vi "allSettings.vi"() -> ()   [LabVIEW 2018]
panel:
  in  "Additional Commands":T1={"Read/Write RAM"={"Dictionary Name"="Enable/Disable Channel", "Dictionary ID"="41", "Update"=FALSE, "Current Data"=""}, "Set/Read Address Pointer"={"Dictionary Name"="Set/Read address pointer", "Dictionary ID"="40", "Update"=FALSE, "Current Data"=""}, "Read EE chksm"={"Dictionary Name"="Read EEPROM Checksum", "Dictionary ID"="42", "Update"=FALSE, "Current Data"=""}, "Hold On/Off"={"Dictionary Name"="Hold On/Off", "Dictionary ID"="43", "Update"=FALSE, "Current Data"=""}, "Emulator Mode"={"Dictionary Name"="Set/Reset Emulator Mode", "Dictionary ID"="44", "Update"=FALSE, "Current Data"=""}, "Write Protect Signal"={"Dictionary Name"="Write Protect Signal On/Off", "Dictionary ID"="45", "Update"=FALSE, "Current Data"=""}}
  in  "Channel Commands":T2={"Chan number"={"Dictionary Name"="Set/Read Channel Number", "Dictionary ID"="30", "Update"=FALSE, "Current Data"=""}, "En/Dis Channel"={"Dictionary Name"="Enable/Disable Channel", "Dictionary ID"="31", "Update"=FALSE, "Current Data"=""}}
  in  "Info Commands":T3={"Part Num"={"Dictionary Name"="Read Part Number", "Dictionary ID"="10", "Update"=FALSE, "Current Data"=""}, "Serial Num"={"Dictionary Name"="Read Part Number", "Dictionary ID"="11", "Update"=FALSE, "Current Data"=""}, "F/W Ver"={"Dictionary Name"="Read F/W & Module Version", "Dictionary ID"="12", "Update"=FALSE, "Current Data"=""}, "Status Byte"={"Dictionary Name"="Read Status Byte", "Dictionary ID"="13", "Update"=FALSE, "Ready/Busy"=FALSE, "Data in FIFO?"=FALSE, "FIFO Full?"=FALSE, "Event Mode On?"=FALSE, "GPIO I/P State"=FALSE, "Parity Error"=FALSE}, "Temp"={"Dictionary Name"="Read Temperature", "Dictionary ID"="14", "Update"=FALSE, "Current Data"=""}}
  in  "C&C Commands":T4={"Send Break"={"Dictionary Name"="Send Break Command", "Dictionary ID"="20", "Update"=FALSE, "Current Data"=""}, "Clear FIFO"={"Dictionary Name"="Clear Event FIFO", "Dictionary ID"="21", "Update"=FALSE, "Current Data"=""}, "Event Mode ON/OFF"={"Dictionary Name"="Event Mode On/Off", "Dictionary ID"="22", "Update"=FALSE, "Current Data"=""}, "Set Energy Threshold"={"Dictionary Name"="Set/Read Energy Threshold", "Dictionary ID"="23", "Update"=FALSE, "Current Data"=""}, "Set GPIO Mode"={"Dictionary Name"="Set/Read GPIO Signal Mode", "Dictionary ID"="24", "Update"=FALSE, "Current Data"=""}, "R/W Clock Freq"={"Dictionary Name"="Read/Write Clock Frequency", "Dictionary ID"="25", "Update"=FALSE, "Current Data"=""}, "Update/Restore Setup"={"Dictionary Name"="Update/Restore Setup", "Dictionary ID"="26", "Update"=FALSE, "Current Data"=""}, "Update/Read Peaking Time"={"Dictionary Name"="Update/Read Peaking Time", "Dictionary ID"="27", "Update"=FALSE, "Current Data"=""}, "Run/Read Self Test"={"Dictionary Name"="Run Self test/ Read Results", "Dictionary ID"="28", "Update"=FALSE, "Current Data"=""}}
  # "Additional Commands"
  # "Channel Commands"
  # "Information Commands"
  # "Configuration & Control Commands"
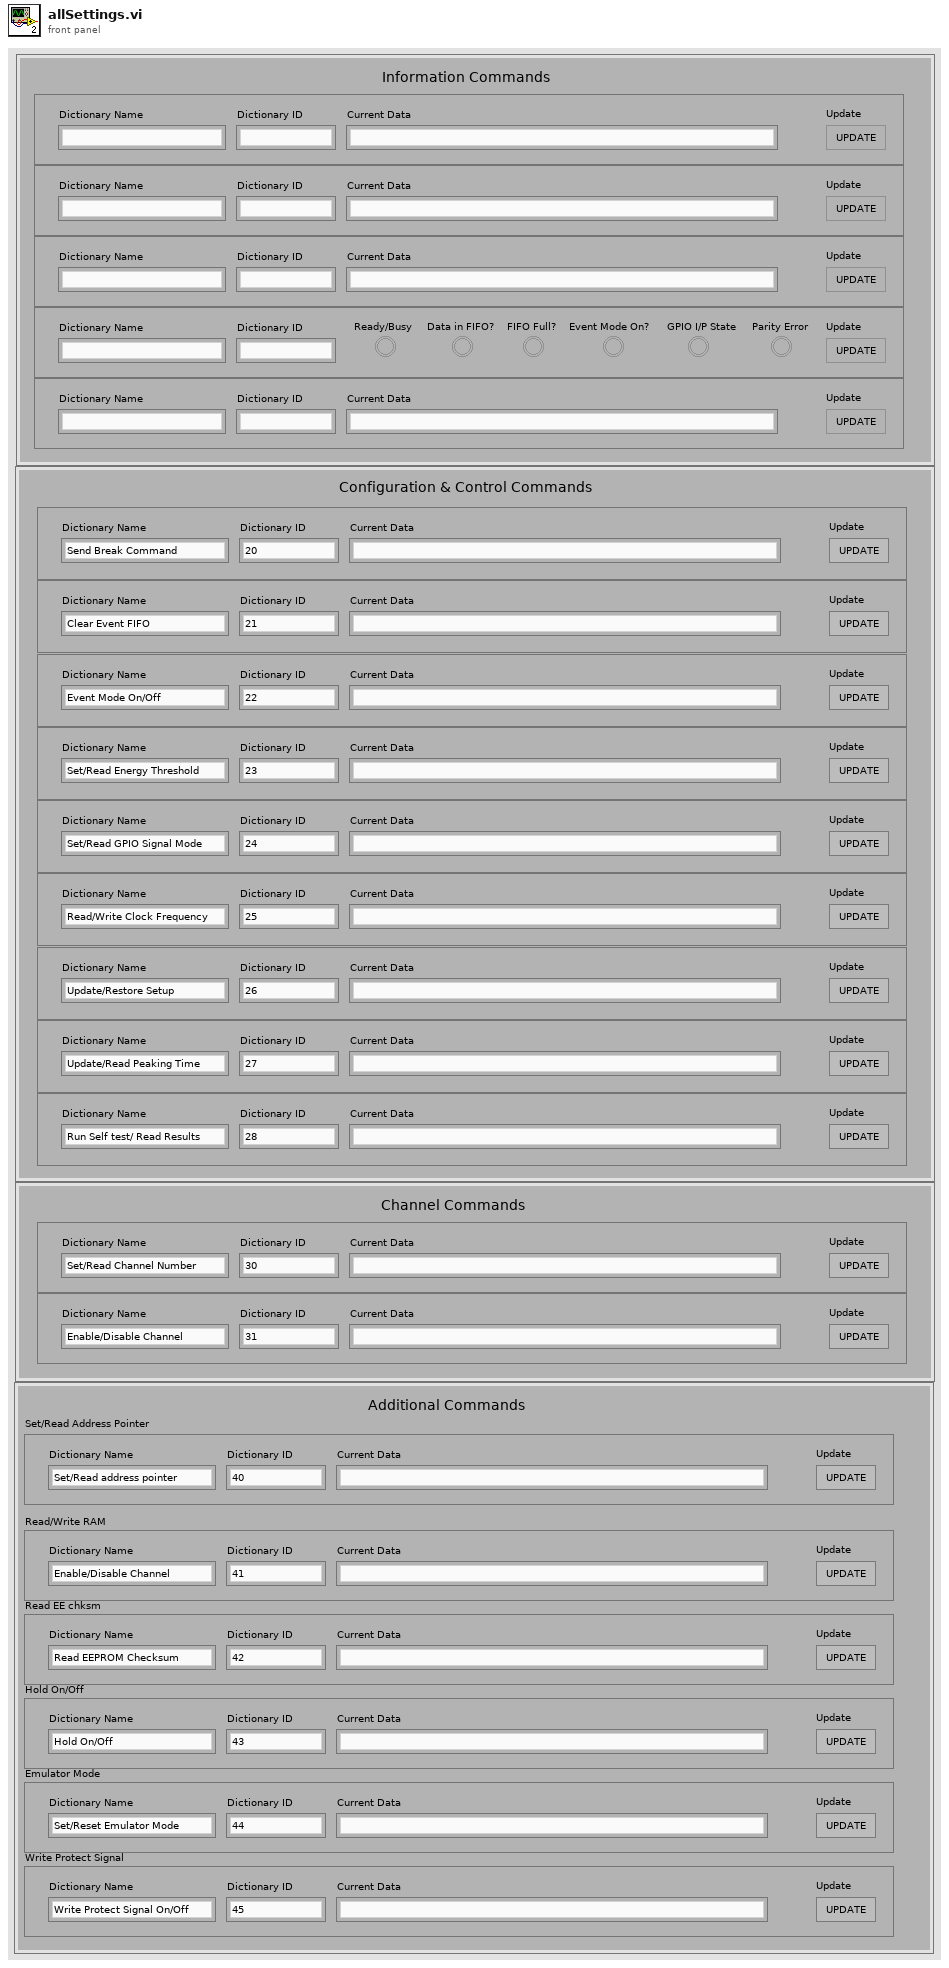
[diagram p1: front panel]
types:
  T1 = cluster{"Read/Write RAM":cluster{"Dictionary Name":string, "Dictionary ID":string, "Update":bool, "Current Data":string}, "Set/Read Address Pointer":cluster{"Dictionary Name":string, "Dictionary ID":string, "Update":bool, "Current Data":string}, "Read EE chksm":cluster{"Dictionary Name":string, "Dictionary ID":string, "Update":bool, "Current Data":string}, "Hold On/Off":cluster{"Dictionary Name":string, "Dictionary ID":string, "Update":bool, "Current Data":string}, "Emulator Mode":cluster{"Dictionary Name":string, "Dictionary ID":string, "Update":bool, "Current Data":string}, "Write Protect Signal":cluster{"Dictionary Name":string, "Dictionary ID":string, "Update":bool, "Current Data":string}}
  T2 = cluster{"Chan number":cluster{"Dictionary Name":string, "Dictionary ID":string, "Update":bool, "Current Data":string}, "En/Dis Channel":cluster{"Dictionary Name":string, "Dictionary ID":string, "Update":bool, "Current Data":string}}
  T3 = cluster{"Part Num":cluster{"Dictionary Name":string, "Dictionary ID":string, "Update":bool, "Current Data":string}, "Serial Num":cluster{"Dictionary Name":string, "Dictionary ID":string, "Update":bool, "Current Data":string}, "F/W Ver":cluster{"Dictionary Name":string, "Dictionary ID":string, "Update":bool, "Current Data":string}, "Status Byte":cluster{"Dictionary Name":string, "Dictionary ID":string, "Update":bool, "Ready/Busy":bool, "Data in FIFO?":bool, "FIFO Full?":bool, "Event Mode On?":bool, "GPIO I/P State":bool, "Parity Error":bool}, "Temp":cluster{"Dictionary Name":string, "Dictionary ID":string, "Update":bool, "Current Data":string}}
  T4 = cluster{"Send Break":cluster{"Dictionary Name":string, "Dictionary ID":string, "Update":bool, "Current Data":string}, "Clear FIFO":cluster{"Dictionary Name":string, "Dictionary ID":string, "Update":bool, "Current Data":string}, "Event Mode ON/OFF":cluster{"Dictionary Name":string, "Dictionary ID":string, "Update":bool, "Current Data":string}, "Set Energy Threshold":cluster{"Dictionary Name":string, "Dictionary ID":string, "Update":bool, "Current Data":string}, "Set GPIO Mode":cluster{"Dictionary Name":string, "Dictionary ID":string, "Update":bool, "Current Data":string}, "R/W Clock Freq":cluster{"Dictionary Name":string, "Dictionary ID":string, "Update":bool, "Current Data":string}, "Update/Restore Setup":cluster{"Dictionary Name":string, "Dictionary ID":string, "Update":bool, "Current Data":string}, "Update/Read Peaking Time":cluster{"Dictionary Name":string, "Dictionary ID":string, "Update":bool, "Current Data":string}, "Run/Read Self Test":cluster{"Dictionary Name":string, "Dictionary ID":string, "Update":bool, "Current Data":string}}
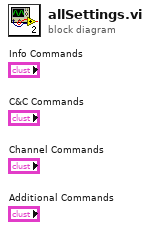
[diagram p0: block diagram]
diagram:
